vi "CloseMIPI_RFFE.vi"(8 "error in (no error)":errorcluster, 9 "Number of Samples":i32, 10 "Data Array":u8[][](array[numeric]), 11 "RFFE_Data":T1 {"Toggle (high to low)" items=["0", "1", "Z", "L", "H", "X", "T", "V"]; "X Array" items=["0", "1", "Z", "L", "H", "X", "T", "V"]; "Z Array" items=["0", "1", "Z", "L", "H", "X", "T", "V"]; "L Array" items=["0", "1", "Z", "L", "H", "X", "T", "V"]; "H Array" items=["0", "1", "Z", "L", "H", "X", "T", "V"]; "One Array" items=["0", "1", "Z", "L", "H", "X", "T", "V"]; "Zero Array" items=["0", "1", "Z", "L", "H", "X", "T", "V"]}) -> (0 "error out":errorcluster, 3 "Digital Waveform":digitalwaveform(waveform))   [LabVIEW 2013]
doc: "This VI converts the 2D data array to Digital Waveform data."
uses:
  Ctrls/RFFE_Data.ctl
  Ctrls/ClockDataChannels.ctl
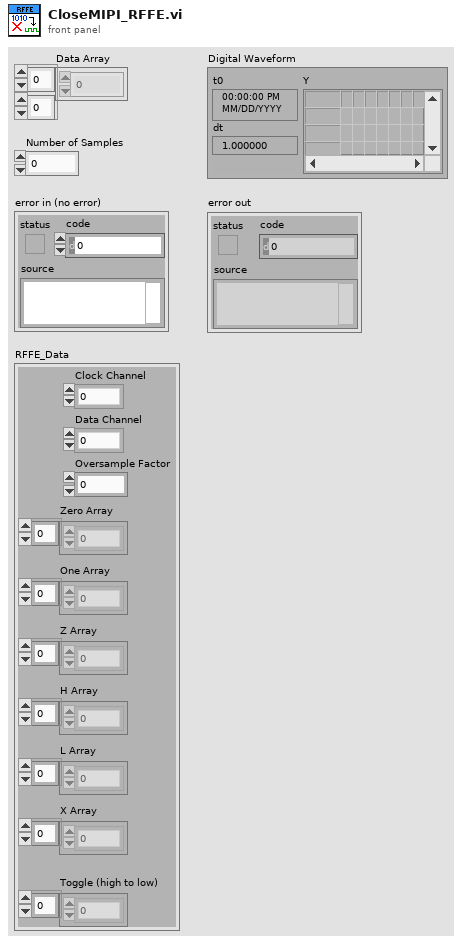
[diagram p1: front panel]
types:
  T1 = typedef "RFFE_Data.ctl" = cluster{"Clock Channel":T2, "Data Channel":T2, "Oversample Factor":u8, "Zero Array":u8[], "One Array":u8[], "Z Array ":u8[], "H Array":u8[], "L Array":u8[], "X Array":u8[], "Toggle (high to low)":u8[]}
  T2 = typedef "ClockDataChannels.ctl" = enum16{"0", "1"}
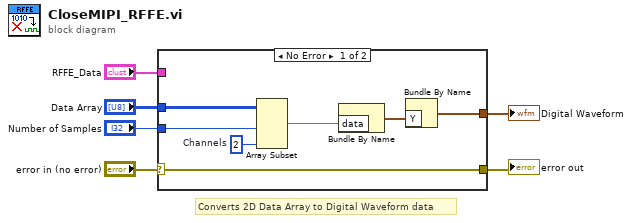
[diagram p0: block diagram]
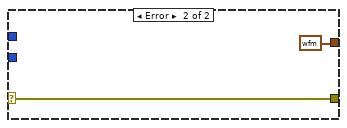
[diagram p2: hidden frame]
diagram:
  # "Converts 2D Data Array to Digital Waveform data"
  n1 = case shown="No Error" "error in (no error)" {
    selector: "error in (no error)" -> [w7 w15]
    tunnel: "Number of Samples" -> [w12 _]
    tunnel: "Data Array" -> [w11 _]
    tunnel: [w9 digitalwaveform {"t0"=timestamp(0 s since 1904-01-01), "dt"=0.0, "Y"={"transitions"=[], "data"=[]}} ("Digital Waveform")] -> w4
    tunnel: [w7 w15] -> w2
    tunnel: "RFFE_Data" -> [_ _]
    frame No Error {
      w10 = 2  # Channels
      n2 = Array Subset(array=w11, length (row)=w12, length (col)=w10) -> (w13:u8[][])  [unwired: 2 in]
      n3 = Bundle By Name("data"=w13) -> (w8:digitaldata)  [unwired: 1 in]
      n4 = Bundle By Name("Y"=w8) -> (w9:digitalwaveform)  [unwired: 1 in]
    }
    frame Error {
    }
  }
  "error out" <- w2
  "Digital Waveform" <- w4
